vi "Parse Path String.vi"(0 "Path in":string, 2 "String Separator (:)":string=":") -> (4 "Folder Hierarchy":string[](array[string]), 5 "File/Folder":string)   [LabVIEW 2019]
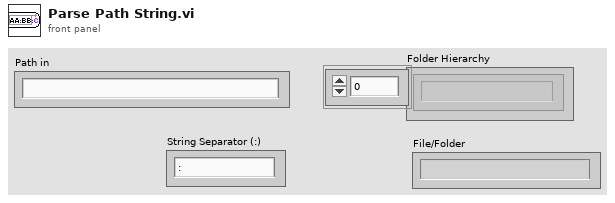
[diagram p1: front panel]
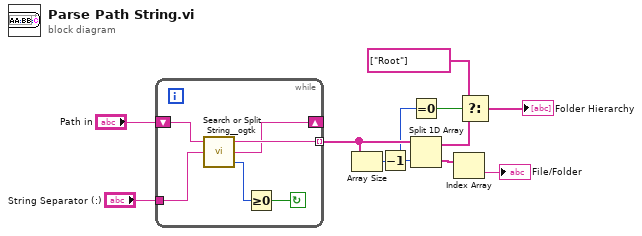
[diagram p0: block diagram]
diagram:
  n1 = while {
    tunnel: "String Separator (:)" -> [w16]
    shift-right: [w12] -> _
    shift-left: "Path in" -> [w17]
    tunnel: [w14] -> w8 mode=indexing
    stop <- w13 continue-if-true
    n2 = call <userlib>:"Search or Split String__ogtk.vi"("search string/char (-)"=w16, "string"=w17) -> ("offset after match"=w15:i32, "substring after match"=w12:string, "substring before match"=w14:string)  [unwired: 1 in]
    n3 = Greater Or Equal To 0?(x=w15) -> (x >= 0?=w13:bool)
  }
  n4 = Array Size(array=w8) -> (size(s)=w9:i32)
  n5 = Decrement(x=w9) -> (x-1=w5:i32)
  n6 = Equal To 0?(x=w5) -> (x = 0?=w4:bool)
  n7 = Split 1D Array(array=w8, index=w5) -> (first subarray=w3:string[], second subarray=w6:string[])
  n8 = Index Array(array=w6) -> (element=→"File/Folder":string)  [unwired: 1 in]
  n9 = Select(t=string[] ["Root"], s=w4, f=w3) -> (s? t:f=→"Folder Hierarchy":string[])
